vi "Teleop.vi"(10 "Match Info":T1={"Autonomous Elapsed Seconds"=0.0, "TeleOp Elapsed Seconds"=0.0, "Disabled Elapsed Seconds"=0.0, "Visited Autonomous"=FALSE, "Visited TeleOp"=FALSE, "Visited Disabled"=FALSE, "Autonomous Settings"={"Autonomous Style"=enum."Independent", "VI Refnum"=refnum}}, 11 "Call Context":T2) -> ()   [LabVIEW 2013]
doc: "This VI is called for each TeleOp packet received from the DS where the robot is not disabled. It is often used to read from the joysticks and update I/O or to update setpoints for timed control loops. It should complete and return within 20 milliseconds or it may miss DS packets."
uses:
  <vilib>/Rock Robotics/WPI/DriverStation/WPI_DriverStationDerivedRobotMode.ctl
  <vilib>/Rock Robotics/WPI/DriverStation/WPI_DriverStationMatch Info.ctl
  <vilib>/Rock Robotics/WPI/Solenoid/WPI_SolenoidValue.ctl
  Robot Global Data.vi
  Gyro/Gyro Global.vi
  <vilib>/Rock Robotics/WPI/Joystick/WPI_JoystickGetSetRefNum.vi
  <vilib>/Rock Robotics/WPI/Solenoid/WPI_SolenoidSetEnum.vi
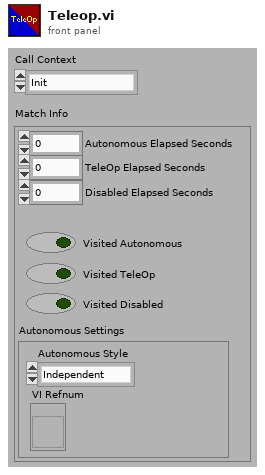
[diagram p1: front panel]
types:
  T1 = typedef "WPI_DriverStationMatch Info.ctl" = cluster{"Autonomous Elapsed Seconds":dbl, "TeleOp Elapsed Seconds":dbl, "Disabled Elapsed Seconds":dbl, "Visited Autonomous":bool, "Visited TeleOp":bool, "Visited Disabled":bool, "Autonomous Settings":cluster{"Autonomous Style":enum16{"Iterative", "Independent"}, "VI Refnum":refnum<vi>}}
  T2 = typedef "WPI_DriverStationDerivedRobotMode.ctl" = enum16{"Init", "Execute", "Stop"}
  T3 = typedef "WPI_JoystickDevRef.ctl" = cluster{"Device":T4}
  T4 = typedef "WPI_JoystickDeviceEnum.ctl" = enum16{"USB 1", "USB 2", "USB 3", "USB 4", "Kinect 1", "Kinect 2"}
  T5 = typedef "WPI_JoystickButtonState.ctl" = cluster{"Button 1":bool, "Button 2":bool, "Button 3":bool, "Button 4":bool, "Button 5":bool, "Button 6":bool, "Button 7":bool, "Button 8":bool, "Button 9":bool, "Button 10":bool, "Button 11":bool, "Button 12":bool}
  T6 = cluster{"axis 1 (x)":dbl, "axis 2 (y)":dbl, "axis 3 (throttle)":dbl, "axis 4":dbl, "axis 5":dbl, "axis 6":dbl}
  T7 = typedef "WPI_GyroDevRef.ctl" = cluster{"DevStatus":errorcluster, "Analog Module":T8, "Analog Channel":T9, "Offset":dbl, "Gain (VoltsPerDegree/Second)":dbl}
  T8 = typedef "FPGA_TypedefAnalogModule.ctl" = enum16{"Analog Module 1", "Analog Module 2"}
  T9 = typedef "FPGA_AIChannel.ctl" = enum8{"AI 1", "AI 2", "AI 3", "AI 4", "AI 5", "AI 6", "AI 7", "AI 8", "Invalid"}
  T10 = enum16{"Wait", "Clear", "Release", "Cock", "Reset"}
  T11 = typedef "WPI_DigitalInputDevRef.ctl" = cluster{"DevStatus":errorcluster, "DIO Channel":T12, "Digital Module":T13}
  T12 = typedef "FPGA_DIOChannel.ctl" = enum8{"DIO 1", "DIO 2", "DIO 3", "DIO 4", "DIO 5", "DIO 6", "DIO 7", "DIO 8", "DIO 9", "DIO 10", "DIO 11", "DIO 12", "DIO 13", "DIO 14", "Invalid"}
  T13 = typedef "FPGA_TypedefDigitalModule.ctl" = enum16{"Digital Module 1", "Digital Module 2"}
  T14 = typedef "WPI_SolenoidValue.ctl" = enum16{"Off", "On", "Forward", "Reverse"}
  T15 = typedef "WPI_MotorControlDeviceRef.ctl" = cluster{"DeviceStatus":errorcluster, "Type":enum16{"PWM", "CAN"}, "PWM":cluster{"Digital Module":T13, "PWM Channel":T16, "DeadBand":T17}, "CAN":cluster{"Device Number":u8, "Control Mode":T18, "Semaphore":T19, "Max Vout":dbl}, "Invert":bool, "TransformRef":T20, "InvTransformRef":T20}
  T16 = typedef "FPGA_DIOPWMChannel.ctl" = enum8{"PWM 1", "PWM 2", "PWM 3", "PWM 4", "PWM 5", "PWM 6", "PWM 7", "PWM 8", "PWM 9", "PWM 10", "Invalid"}
  T17 = typedef "WPI_PWMDeadband.ctl" = cluster{"Name":string, "maxPositivePwm":i32, "minPositivePwm":i32, "centerPwm":i32, "maxNegativePwm":i32, "minNegativePwm":i32, "angularRange":u16}
  T18 = typedef "WPI_CANJaguar_ControlMode.ctl" = enum8{"Percent VBus", "Current", "Speed", "Position", "Voltage"}
  T19 = typedef "Semaphore RefNum" = refnum<k1>
  T20 = typedef "WPI_PWMTransform_ConPane.ctl" = refnum<vi>
  T21 = typedef "WPI_SolenoidDevRef.ctl" = cluster{"DevStatus":errorcluster, "Solenoid Module":T22, "Forward Solenoid Channel":T23, "Reverse Solenoid Channel":T23}
  T22 = typedef "FPGA_TypedefSolenoidModule.ctl" = enum16{"Solenoid Module 1", "Solenoid Module 2"}
  T23 = typedef "WPI_SolenoidChannel.ctl" = enum8{"Solenoid 1", "Solenoid 2", "Solenoid 3", "Solenoid 4", "Solenoid 5", "Solenoid 6", "Solenoid 7", "Solenoid 8", "Invalid"}
  T24 = typedef "WPI_EncoderDevRef.ctl" = cluster{"DevStatus":errorcluster, "EncoderIndex":T25, "CounterIndex":T26, "DistancePerCount":dbl, "Decoding Type":T27}
  T25 = typedef "FPGA_EncoderIdx.ctl" = enum8{"Enc 0", "Enc 1", "Enc 2", "Enc 3", "Invalid"}
  T26 = typedef "FPGA_CounterCtrSystemIndex.ctl" = enum8{"Ctr 0", "Ctr 1", "Ctr 2", "Ctr 3", "Ctr 4", "Ctr 5", "Ctr 6", "Ctr 7", "Invalid"}
  T27 = typedef "WPI_EncoderType.ctl" = enum16{"1x", "2x", "4x"}
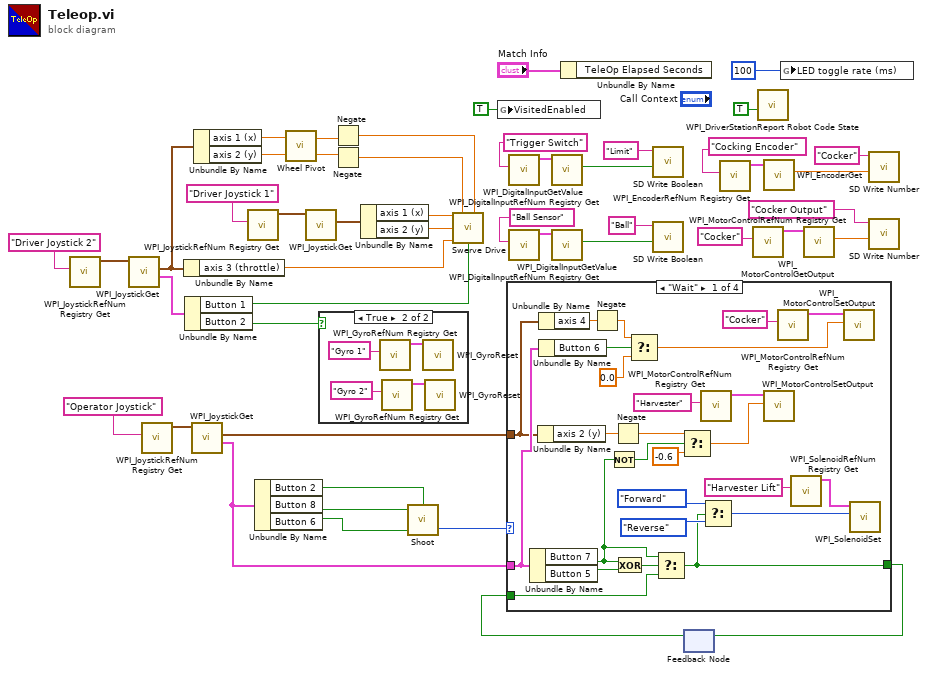
[diagram p0: block diagram]
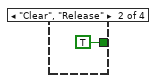
[diagram p2: hidden frame]
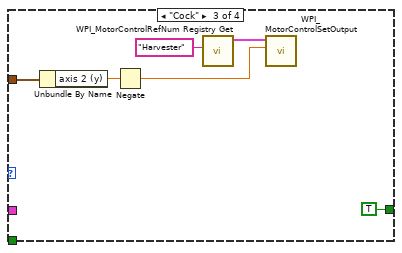
[diagram p3: hidden frame]
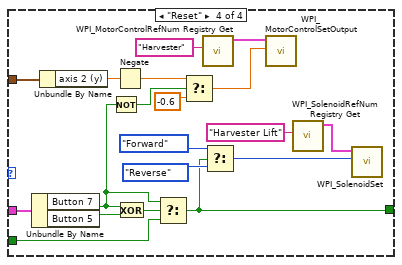
[diagram p4: hidden frame]
diagram:
  n1 = call <vilib>:"WPI_JoystickRefNum Registry Get.vi"("refnum name"="Driver Joystick 2") -> ("JoystickDevRef"=w13:T3)  [unwired: 1 in, 9 out]
  n2 = call <vilib>:"WPI_JoystickGet.vi"("JoystickDevRef"=w13) -> ("Buttons"=w7:T5, "Axes"=w2:T6)  [unwired: 1 in, 4 out]
  n3 = call <vilib>:"WPI_JoystickRefNum Registry Get.vi"("refnum name"="Operator Joystick") -> ("JoystickDevRef"=w45:T3)  [unwired: 1 in, 9 out]
  n4 = Unbundle By Name(w2) -> ("axis 3 (throttle)"=w5:dbl)
  n5 = Unbundle By Name(w7) -> ("Button 1"=w6:bool, "Button 2"=w37:bool)
  n6 = call <vilib>:"WPI_JoystickGet.vi"("JoystickDevRef"=w45) -> ("Buttons"=w43:T5, "Axes"=w19:T6)  [unwired: 1 in, 4 out]
  n7 = Unbundle By Name(w2) -> ("axis 1 (x)"=w12:dbl, "axis 2 (y)"=w11:dbl)
  n8 = call <vilib>:"WPI_JoystickRefNum Registry Get.vi"("refnum name"="Driver Joystick 1") -> ("JoystickDevRef"=w16:T3)  [unwired: 1 in, 9 out]
  n9 = Unbundle By Name(w43) -> ("Button 2"=w38:bool, "Button 8"=w20:bool, "Button 6"=w39:bool)
  n10 = call "Wheel Pivot.vi"("y in"=w11, "x in"=w12) -> ("y out"=w10:dbl, "x out"=w9:dbl)
  n11 = call <vilib>:"WPI_JoystickGet.vi"("JoystickDevRef"=w16) -> ("Axes"=w8:T6)  [unwired: 1 in, 5 out]
  n12 = case shown="True" w37 {
    frame False {
    }
    frame True {
      n13 = call <vilib>:"WPI_GyroRefNum Registry Get.vi"("refnum name"="Gyro 1") -> ("GyroDevRef"=w51:T7)  [unwired: 9 in, 1 out]
      n14 = call <vilib>:"WPI_GyroRefNum Registry Get.vi"("refnum name"="Gyro 2") -> ("GyroDevRef"=w50:T7)  [unwired: 9 in, 1 out]
      n15 = call <vilib>:"WPI_GyroReset.vi"("GyroDevRef"=w51) -> ()  [unwired: 9 in, 2 out]
      n16 = call <vilib>:"WPI_GyroReset.vi"("GyroDevRef"=w50) -> ()  [unwired: 9 in, 2 out]
    }
  }
  n17 = Negate(x=w9) -> (-x=w18:dbl)
  n18 = Negate(x=w10) -> (-x=w17:dbl)
  n19 = Unbundle By Name(w8) -> ("axis 1 (x)"=w4:dbl, "axis 2 (y)"=w3:dbl)
  n20 = call "Shoot.vi"("Reset"=w38, "Safety Override"=w39, "Shoot"=w20) -> ("State"=w42:T10)  [unwired: 1 in, 1 out]
  n21 = call "Swerve Drive.vi"("X"=w4, "Rot. Point Y"=w17, "Rot. Point X"=w18, "Y"=w3, "Z"=w5, "Robot-Centric"=w6) -> ()  [unwired: 10 in]
  n22 = global write "Gyro Global.vi" "VisitedEnabled"(TRUE ("VisitedEnabled")) -> ()
  n23 = call <vilib>:"WPI_DigitalInputRefNum Registry Get.vi"("refnum name"="Trigger Switch") -> ("DigitalInputDevRef"=w36:T11)  [unwired: 9 in, 1 out]
  n24 = call <vilib>:"WPI_DigitalInputRefNum Registry Get.vi"("refnum name"="Ball Sensor") -> ("DigitalInputDevRef"=w29:T11)  [unwired: 9 in, 1 out]
  n25 = call <vilib>:"WPI_DigitalInputGetValue.vi"("DigitalInputDevRef"=w36) -> ("Value"=w34:bool)  [unwired: 8 in, 2 out]
  n26 = call <vilib>:"WPI_DigitalInputGetValue.vi"("DigitalInputDevRef"=w29) -> ("Value"=w31:bool)  [unwired: 8 in, 2 out]
  n27 = Unbundle By Name("Match Info") -> ()  [unwired: 1 out]
  n28 = call <vilib>:"SD Write Boolean.vi"("Boolean"=w34, "Name"="Limit") -> ()  [unwired: 8 in, 2 out]
  n29 = call <vilib>:"SD Write Boolean.vi"("Boolean"=w31, "Name"="Ball") -> ()  [unwired: 8 in, 2 out]
  n30 = feedback #1() -> (w40:bool)  [unwired: 1 in]
  n31 = case shown="\"Wait\"" w42 {
    tunnel: w43 -> [w59 _ _ w104]
    tunnel: [w68 TRUE ("Button 7") TRUE ("Button 7") w92] -> w41
    tunnel: w40 -> [w76 _ _ w101]
    tunnel: w19 -> [w54 _ w84 w94]
    frame "Wait" {
      n32 = Unbundle By Name(w59) -> ("Button 7"=w66:bool, "Button 5"=w78:bool)
      n33 = Unbundle By Name(w54) -> ("axis 2 (y)"=w67:dbl)
      n34 = Unbundle By Name(w54) -> ("axis 4"=w57:dbl)
      n35 = Unbundle By Name(w59) -> ("Button 6"=w58:bool)
      n36 = Negate(x=w57) -> (-x=w53:dbl)
      n37 = Not(x=w66) -> (.not. x?=w65:bool)
      n38 = Negate(x=w67) -> (-x=w62:dbl)
      n39 = Exclusive Or(1:w78, 2:w66) -> (0:w77:bool)
      n40 = Select(t=w53, s=w58, f=0.0) -> (s? t:f=w55:dbl)
      n41 = Select(t=w66, s=w77, f=w76) -> (s? t:f=w68:bool)
      n42 = Select(t=w62, s=w65, f=-0.6) -> (s? t:f=w63:dbl)
      n43 = call <vilib>:"WPI_MotorControlRefNum Registry Get.vi"("refnum name"="Harvester") -> ("MotorControlDevRef"=w69:T15)  [unwired: 9 in, 1 out]
      n44 = Select(t=WPI_SolenoidValue."Forward" ("Value"), s=w68, f=WPI_SolenoidValue."Reverse" ("Value")) -> (s? t:f=w73:T14)
      n45 = call <vilib>:"WPI_MotorControlSetOutput.vi"("Output"=w63, "MotorControlDevRef"=w69) -> ()  [unwired: 7 in, 3 out]
      n46 = call <vilib>:"WPI_MotorControlRefNum Registry Get.vi"("refnum name"="Cocker") -> ("MotorControlDevRef"=w60:T15)  [unwired: 9 in, 1 out]
      n47 = call <vilib>:"WPI_SolenoidRefNum Registry Get.vi"("refnum name"="Harvester Lift") -> ("SolenoidDevRef"=w72:T21)  [unwired: 9 in, 1 out]
      n48 = call <vilib>:"WPI_MotorControlSetOutput.vi"("Output"=w55, "MotorControlDevRef"=w60) -> ()  [unwired: 7 in, 3 out]
      n49 = call-poly <vilib>:"WPI_SolenoidSet.vi"("Value"=w73, "SolenoidDevRef"=w72) -> ()  [unwired: 8 in, 2 out]
    }
    frame "Clear", "Release" {
    }
    frame "Cock" {
      n50 = Unbundle By Name(w84) -> ("axis 2 (y)"=w82:dbl)
      n51 = Negate(x=w82) -> (-x=w80:dbl)
      n52 = call <vilib>:"WPI_MotorControlRefNum Registry Get.vi"("refnum name"="Harvester") -> ("MotorControlDevRef"=w83:T15)  [unwired: 9 in, 1 out]
      n53 = call <vilib>:"WPI_MotorControlSetOutput.vi"("Output"=w80, "MotorControlDevRef"=w83) -> ()  [unwired: 7 in, 3 out]
    }
    frame "Reset" {
      n54 = Unbundle By Name(w104) -> ("Button 7"=w90:bool, "Button 5"=w103:bool)
      n55 = Unbundle By Name(w94) -> ("axis 2 (y)"=w91:dbl)
      n56 = Not(x=w90) -> (.not. x?=w89:bool)
      n57 = Negate(x=w91) -> (-x=w86:dbl)
      n58 = Exclusive Or(1:w103, 2:w90) -> (0:w102:bool)
      n59 = Select(t=w90, s=w102, f=w101) -> (s? t:f=w92:bool)
      n60 = Select(t=w86, s=w89, f=-0.6) -> (s? t:f=w87:dbl)
      n61 = call <vilib>:"WPI_MotorControlRefNum Registry Get.vi"("refnum name"="Harvester") -> ("MotorControlDevRef"=w93:T15)  [unwired: 9 in, 1 out]
      n62 = Select(t=WPI_SolenoidValue."Forward" ("Value"), s=w92, f=WPI_SolenoidValue."Reverse" ("Value")) -> (s? t:f=w98:T14)
      n63 = call <vilib>:"WPI_MotorControlSetOutput.vi"("Output"=w87, "MotorControlDevRef"=w93) -> ()  [unwired: 7 in, 3 out]
      n64 = call <vilib>:"WPI_SolenoidRefNum Registry Get.vi"("refnum name"="Harvester Lift") -> ("SolenoidDevRef"=w97:T21)  [unwired: 9 in, 1 out]
      n65 = call-poly <vilib>:"WPI_SolenoidSet.vi"("Value"=w98, "SolenoidDevRef"=w97) -> ()  [unwired: 8 in, 2 out]
    }
  }
  n66 = feedback-in #1(w41) -> ()
  n67 = call <vilib>:"WPI_EncoderRefNum Registry Get.vi"("refnum name"="Cocking Encoder") -> ("EncoderDevRef"=w28:T24)  [unwired: 9 in, 1 out]
  n68 = call <vilib>:"WPI_MotorControlRefNum Registry Get.vi"("refnum name"="Cocker") -> ("MotorControlDevRef"=w23:T15)  [unwired: 9 in, 1 out]
  n69 = call <vilib>:"WPI_DriverStationReport Robot Code State.vi"("TeleOp"=TRUE ("Autonomous")) -> ()  [unwired: 10 in, 1 out]
  n70 = call <vilib>:"WPI_EncoderGet.vi"("EncoderDevRef"=w28) -> ("Distance"=w26:dbl)  [unwired: 5 in, 5 out]
  n71 = global write "Robot Global Data.vi" "LED toggle rate (ms)"(u32 100 ("LED ms toggle rate")) -> ()
  n72 = call <vilib>:"WPI_MotorControlGetOutput.vi"("MotorControlDevRef"=w23) -> ("Output"=w22:dbl)  [unwired: 8 in, 2 out]
  n73 = call <vilib>:"SD Write Number.vi"("Numeric"=w26, "Name"="Cocker") -> ()  [unwired: 8 in, 2 out]
  n74 = call <vilib>:"SD Write Number.vi"("Numeric"=w22, "Name"="Cocker Output") -> ()  [unwired: 8 in, 2 out]
